vi "Version Number to Text.vi"(11 "Version Number":T1) -> (3 "Version Text":string)   [LabVIEW 2016, in "Packages.lvlib"]
uses:
  Packages.lvlib
  Version Number--cluster.ctl
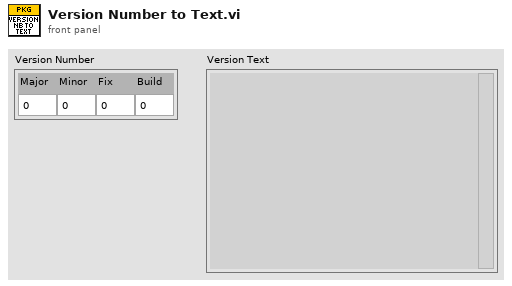
[diagram p1: front panel]
types:
  T1 = typedef "Packages.lvlib/Version Number--cluster.ctl" = cluster{"Major":i32, "Minor":i32, "Fix":i32, "Build":i32}
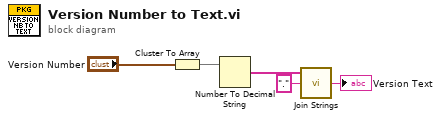
[diagram p0: block diagram]
diagram:
  n1 = Cluster To Array(cluster="Version Number") -> (array=w4:i32[])
  n2 = Number To Decimal String(number=w4) -> (decimal integer string=w3:string[])  [unwired: 1 in]
  n3 = call <vilib>:"Join Strings.vi"("Separator (,)"=".", "Strings In"=w3) -> ("String"=→"Version Text":string)  [unwired: 1 in]
